vi "Heat Orientation.vi"(10 "Direction":T1) -> ()   [LabVIEW 2021, in "Board_Game.lvclass"]
uses:
  Board_Game.lvclass
  Direction.ctl
  Board_Game.lvclass/Board_Game.ctl
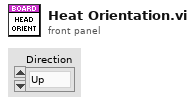
[diagram p1: front panel]
types:
  T1 = typedef "Direction.ctl" = enum16{"Up", "Down", "Left", "Right"}
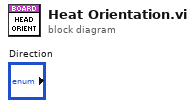
[diagram p0: block diagram]
diagram:
